vi "HostControl_Main.vi"() -> ()   [LabVIEW 2013]
uses:
  Support VIs/operationModes.ctl
  <vilib>/MakerHub/KinectOne/Private/Type Defs/BodyData.ctl
  <vilib>/MakerHub/KinectOne/Private/Type Defs/ClippedEdges.ctl
  <vilib>/MakerHub/KinectOne/Private/Type Defs/HandLeftConfidence.ctl
  <vilib>/MakerHub/KinectOne/Private/Type Defs/HandLeftState.ctl
  <vilib>/MakerHub/KinectOne/Private/Type Defs/HandRightConfidence.ctl
  <vilib>/MakerHub/KinectOne/Private/Type Defs/HandRightState.ctl
  Microsoft.Kinect
  <vilib>/MakerHub/KinectOne/Private/Type Defs/LeanTrackingState.ctl
  Messages.ctl
  Support VIs/messageTypes.ctl
  GainsTDef.ctl
  Support VIs/speeds.ctl
  PolarCoordTdef.ctl
  StopTDef.ctl
  Support VIs/setpointCluster.ctl
  <vilib>/MakerHub/PS4-Controller/Public/Open First Controller.vi
  <vilib>/MakerHub/KinectOne/Private/Initialize Image [Color].vi
  <vilib>/MakerHub/KinectOne/Private/kinectRead [ColorFrame].vi
  <vilib>/MakerHub/KinectOne/Private/kinectRead [BodyFrame].vi
  <vilib>/MakerHub/KinectOne/KinectOne.lvlib
  <vilib>/MakerHub/PS4-Controller/LMH-PS4.lvlib
panel:
  in  "colour mode (T = dist, F = sphere)":bool
  out "Detected Colour":u32(colorbox)
  out "Tracked?":bool
  in  "Forward Speed Limit [rad/s] (10 r/s)":dbl(knob)=2.995028509599303 scale=0.0..10.0
  out "Gains Closed":bool
  out "Setpoint Grtr Closed":bool
  out "Stopper Closed":bool
  out "Kinect Closed":bool
  out "Ctrl Event Loop Off":bool
  out "Controller Off":bool
  out "Hand Ctrl Closed":bool
  out "Message Sender Closed":bool
  in  "ControllerStop":bool
  out "Controller?":bool
  out "Toggle":bool
  in  "Cancel Button":bool
  out "TX":bool
  in  "bodyData":T1[](array[typedef])
  in  "Modulus SP":dbl=1.8
  in  "Reference Colour":u32(colorbox)
  in  "Argument SP":dbl
  out "index":i32
  in  "Operation Mode":T8=1 items=["TeleOp", "Desperate", "ColourMatch"]
  out "Image":T9(plugin-control)
  in  "Kd-Argument":dbl
  in  "Kc-Argument":dbl=0.3
  in  "Kd-Modulus":dbl
  in  "Kc-Modulus":dbl=0.5
  out "Mod":dbl
  out "Arg":dbl
  in  "IT'S TIME TO":bool
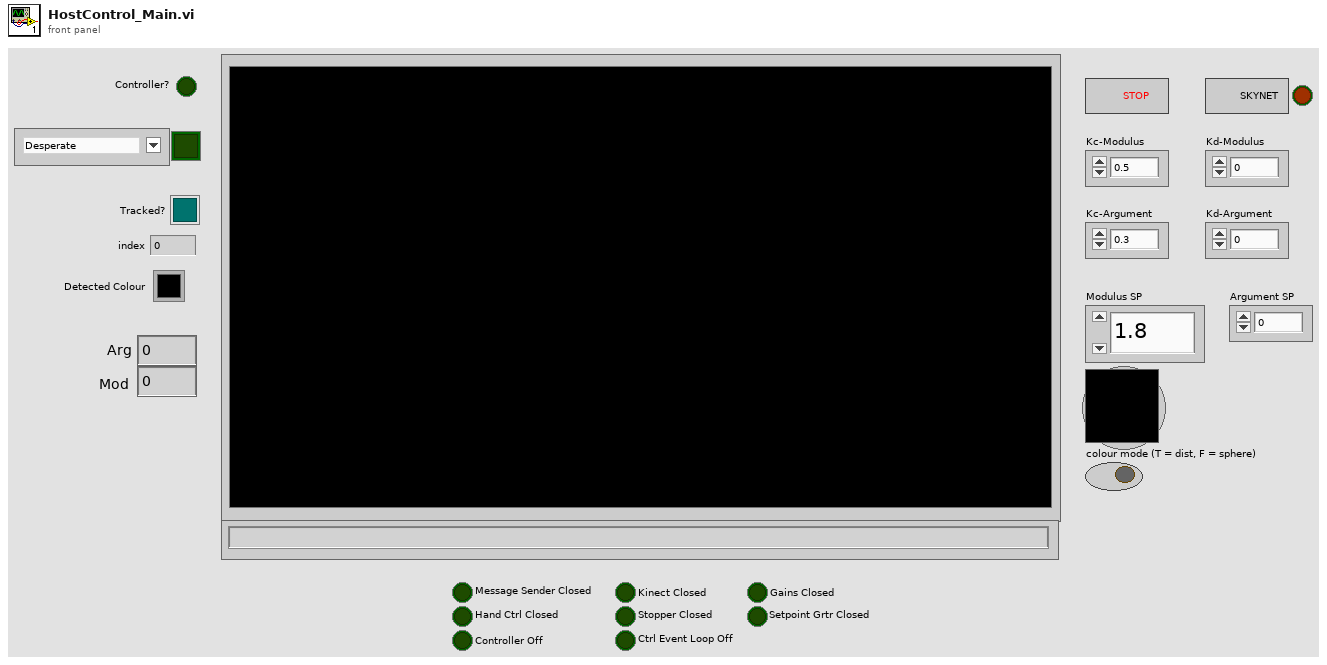
[diagram p1: front panel]
types:
  T1 = typedef "KinectOne.lvlib/BodyData.ctl" = cluster{"ClippedEdges":T2, "HandLeftConfidence":T3, "HandLeftState":T4, "HandRightConfidence":T5, "HandRightState":T6, "IsRestricted":bool, "IsTracked":bool, "JointOrientations":refnum<k24>, "Joints":refnum<k24>, "Lean":refnum<k24>, "LeanTrackingState":T7, "TrackingId":u64}
  T2 = typedef "KinectOne.lvlib/ClippedEdges.ctl" = enum16{"None", "Right", "Left", "Top", "Bottom"}
  T3 = typedef "KinectOne.lvlib/HandLeftConfidence.ctl" = enum16{"Low", "High"}
  T4 = typedef "KinectOne.lvlib/HandLeftState.ctl" = enum16{"Unknown", "NotTracked", "Open", "Closed", "Lasso"}
  T5 = typedef "KinectOne.lvlib/HandRightConfidence.ctl" = enum16{"Low", "High"}
  T6 = typedef "KinectOne.lvlib/HandRightState.ctl" = enum16{"Unknown", "NotTracked", "Open", "Closed", "Lasso"}
  T7 = typedef "KinectOne.lvlib/LeanTrackingState.ctl" = enum16{"NotTracked", "Inferred", "Tracked"}
  T8 = typedef "operationModes.ctl" = u16
  T9 = typedef "IMAQ Image.ctl" = refnum<image>
  T10 = typedef "GainsTDef.ctl" = cluster{"Kc-Modulus":dbl, "Kd-Modulus":dbl, "Kc-Argument":dbl, "Kd-Argument":dbl}
  T11 = typedef "Messages.ctl" = cluster{"message data":variant, "message type":T12}
  T12 = typedef "messageTypes.ctl" = enum16{"Speeds", "Stop", "PolarCoordinates", "Gains", "Setpoints"}
  T13 = typedef "KinectOne.lvlib/KinectSensor References.ctl" = cluster{"KinectSensor":refnum<k24>, "MultiSourceFrameReader":refnum<k24>, "BodyFrameDataInterface":refnum<k24>}
  T14 = typedef "LMH-PS4.lvlib/PS4 Controller Ref.ctl" = cluster{"Controller Ref":refnum<k1>, "PS4 Events Ref":refnum<event-registration>, "Worker Ref":refnum<vi>}
  T15 = typedef "StopTDef.ctl" = cluster{"stop":bool}
  T16 = typedef "speeds.ctl" = cluster{"left motor [rad/s]":dbl, "right motor [rad/s]":dbl}
  T17 = typedef "PolarCoordTdef.ctl" = cluster{"Argument":dbl, "Modulus":dbl, "trackedState":bool}
  T18 = typedef "KinectOne.lvlib/Joint Position.ctl" = cluster{"Camera Space":cluster{"X":dbl, "Y":dbl, "Z":dbl}, "Color Space":cluster{"X":dbl, "Y":dbl}, "Depth Space":cluster{"X":dbl, "Y":dbl}, "Tracking State":enum16{"NotTracked", "Inferred", "Tracked"}}
  T19 = typedef "setpointCluster.ctl" = cluster{"Modulus Setpoint":dbl, "Argument Setpoint":dbl}
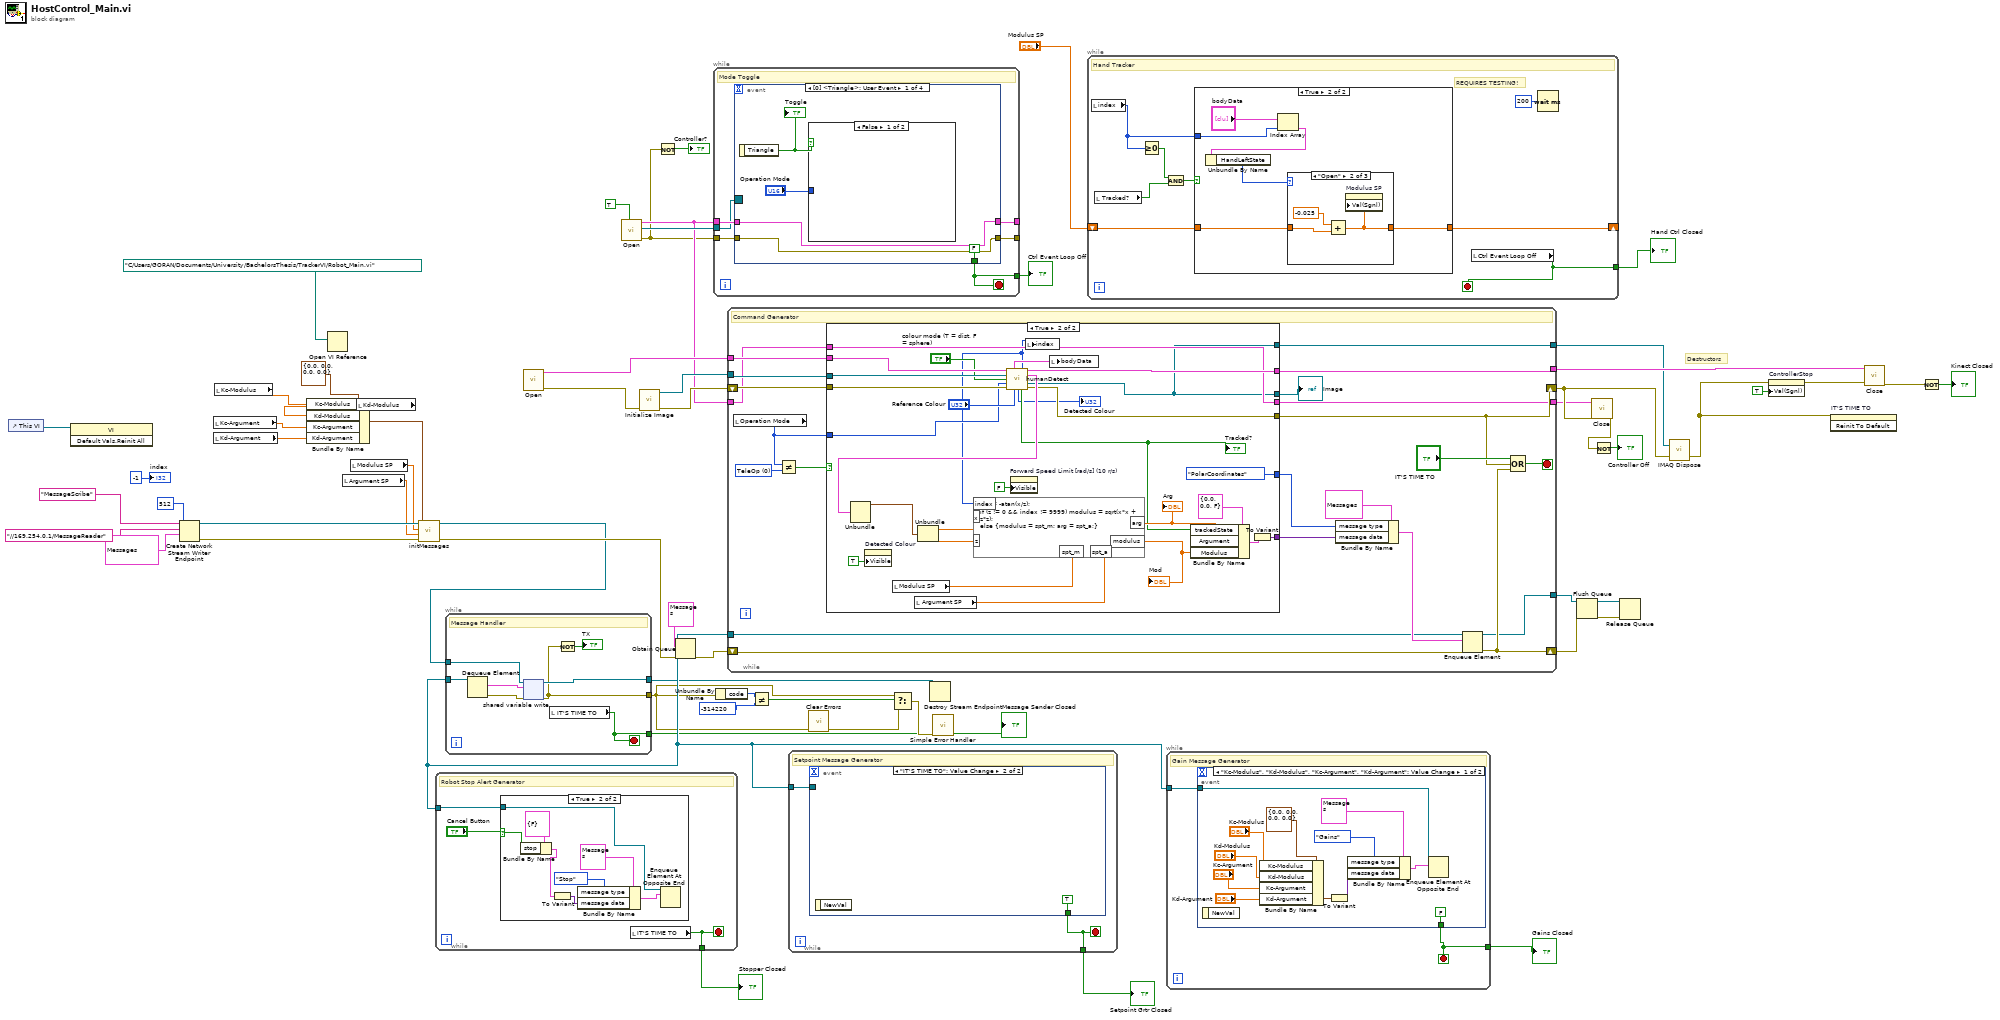
[diagram p0: block diagram]
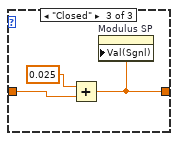
[diagram p4: hidden frame]
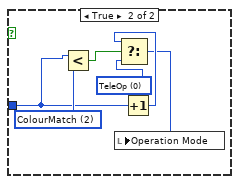
[diagram p5: hidden frame]
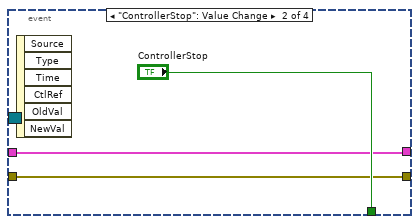
[diagram p6: hidden frame]
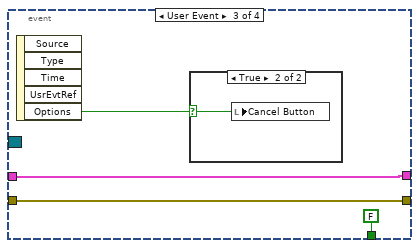
[diagram p7: hidden frame]
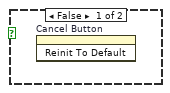
[diagram p8: hidden frame]
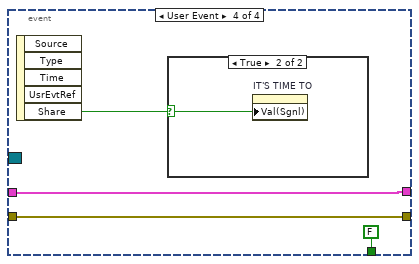
[diagram p9: hidden frame]
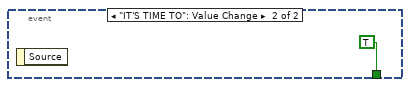
[diagram p12: hidden frame]
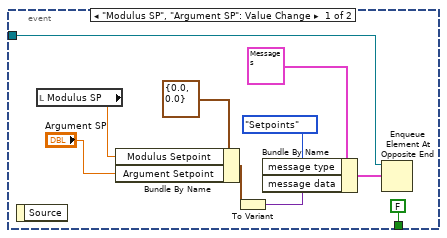
[diagram p13: hidden frame]
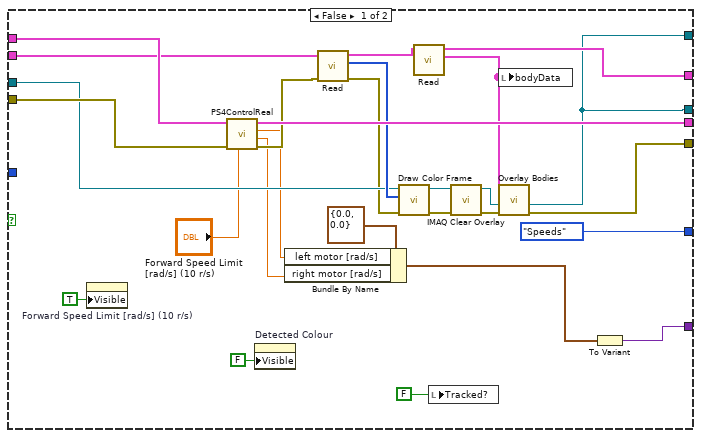
[diagram p14: hidden frame]
diagram:
  # "Destructors"
  n1 = control-ref of="This VI"() -> (w4:refnum<vi>)
  n2 = invoke class="VI" method="Default Vals.Reinit All"(reference=w4) -> ()  [unwired: 2 in, 3 out]
  n3 = Create Network Stream Writer Endpoint(7:512 ("writer buffer size"), 9:T11 {"message data"=variant, "message type"=enum."Setpoints"} ("message"), 10:"//169.254.0.1/MessageReader" ("reader url"), 11:"MessageScribe" ("writer name")) -> (0:w25:errorcluster, 3:w26:refnum<k21>)  [unwired: 3 in]
  n4 = local read "Kc-Argument"() -> (w29:dbl)
  n5 = local read "Kd-Argument"() -> (w28:dbl)
  n6 = local read "Kc-Modulus"() -> (w31:dbl)
  n7 = Open VI Reference(vi path=path "C:/Users/GORAN/Documents/University/BachelorsThesis/TrackerVI/Robot_Main.vi") -> ()  [unwired: 5 in, 2 out]
  n8 = local read "Argument SP"() -> (w23:dbl)
  n9 = local read "Modulus SP"() -> (w24:dbl)
  n10 = local read "Kd-Modulus"() -> (w30:dbl)
  n11 = Bundle By Name(cluster=T10 {"Kc-Modulus"=0.0, "Kd-Modulus"=0.0, "Kc-Argument"=0.0, "Kd-Argument"=0.0}, "Kc-Modulus"=w31, "Kd-Modulus"=w30, "Kc-Argument"=w29, "Kd-Argument"=w28) -> (w27:T10)
  n12 = call "initMessages.vi"("GainsCluster"=w27, "error in (no error)"=w25, "Argument Setpoint"=w23, "Modulus Setpoint"=w24, "writer name in"=w26) -> ("error out"=w22:errorcluster, "Refnum out"=w21:refnum<k21>)  [unwired: 5 in]
  n13 = call <vilib>:"Open.vi"() -> ("Error Out"=w60:errorcluster, "KinectSensor References out"=w52:T13)  [unwired: 10 in]
  n14 = call-poly <vilib>:"Open.vi"("Enable Events (T)"=TRUE) -> ("Error Out"=w20:errorcluster, "Event Registration Refnum"=w53:refnum<event-registration>, "PS4 Controller Ref"=w51:T14)  [unwired: 8 in]
  n15 = call-poly <vilib>:"Initialize Image.vi"("Error In"=w60) -> ("Error Out"=w59:errorcluster, "Color Image"=w58:T9)  [unwired: 9 in]
  n16 = Not(x=w20) -> (.not. x?=→"Controller?":bool)
  n17 = Obtain Queue(element data type=T11 {"message data"=variant, "message type"=enum."Stop"} ("message"), error in (no error)=w22) -> (queue out=w49:refnum<queue>, error out=w56:errorcluster)  [unwired: 3 in, 1 out]
  n18 = while {
    tunnel: w49 -> [w63]
    tunnel: [w61] -> w7
    stop <- w61 stop-if-true
    # "Robot Stop Alert Generator"
    n19 = case shown="True" "Cancel Button" {
      selector: "Cancel Button" -> [_ w66]
      tunnel: w63 -> [_ w67]
      frame False {
      }
      frame True {
        n20 = Bundle By Name(cluster=T15 {"stop"=FALSE} ("Cluster"), "stop"=w66) -> (w64:T15)
        n21 = To Variant(anything=w64) -> (Variant=w70:variant)
        n22 = Bundle By Name(cluster=T11 {"message data"=variant, "message type"=enum."Stop"} ("message"), "message type"=messageTypes."Stop", "message data"=w70) -> (w69:T11)
        n23 = Enqueue Element At Opposite End(queue=w67, element=w69) -> ()  [unwired: 2 in, 3 out]
      }
    }
    n24 = local read "IT'S TIME TO"() -> (w61:bool)
  }
  "Stopper Closed" <- w7
  n25 = while {
    tunnel: w49 -> [w79]
    tunnel: [w76] -> w34
    tunnel: [w75] -> w33
    tunnel: w21 -> [w73]
    tunnel: [w72] -> w8
    stop <- w72 stop-if-true
    # "Message Handler"
    n26 = Dequeue Element(queue=w79) -> (element=w78:T11, error out=w77:errorcluster)  [unwired: 2 in, 2 out]
    n27 = shared-variable-write(w73, w77, w78) -> (w76:refnum<k21>, w75:errorcluster)  [unwired: 1 in, 1 out]
    n28 = local read "IT'S TIME TO"() -> (w72:bool)
    n29 = Not(x=w75) -> (.not. x?=→"TX":bool)
  }
  "Message Sender Closed" <- w8
  n30 = while {
    tunnel: w53 -> [w83]
    tunnel: w20 -> [w84]
    tunnel: [w81] -> _
    tunnel: w51 -> [w85]
    tunnel: [w82] -> _
    tunnel: [w80] -> w9
    stop <- w80 stop-if-true
    # "Mode Toggle"
    n31 = event shown="[0] <Triangle>: User Event" {
      selector: w83 -> [_ _ _ _]
      dyn-events: _ -> [_ _ _ _]
      timeout: _ -> [_ _ _ _]
      tunnel: w85 -> [w88 w98 w102 w107]
      tunnel: w84 -> [w87 w97 w101 w106]
      tunnel: [w88 w98 w102 w107] -> w82
      tunnel: [w87 w97 w101 w106] -> w81
      tunnel: [FALSE ("ControllerStop") "ControllerStop" FALSE ("ControllerStop") FALSE ("ControllerStop")] -> w80
      event User Event {
        n32 = event-data() -> ("Triangle"=w90:bool)  [unwired: 1 in]
        "Toggle" <- w90
        n33 = case shown="False" w90 {
          tunnel: "Operation Mode" -> [_ w91]
          frame False {
          }
          frame True {
            w92 = T8 2 items=["TeleOp", "Desperate", "ColourMatch"] ("Operation Mode 2")
            w93 = T8 0 items=["TeleOp", "Desperate", "ColourMatch"] ("Operation Mode 2")
            n34 = Less?(x=w91, y=w92) -> (x < y?=w96:bool)
            n35 = Increment(x=w91) -> (x+1=w95:T8)
            n36 = Select(t=w95, s=w96, f=w93) -> (s? t:f=w94:T8)
            n37 = local write "Operation Mode"(w94) -> ()
          }
        }
      }
      event "ControllerStop": Value Change {
        n38 = event-data() -> ()  [unwired: 1 in, 6 out]
      }
      event User Event {
        n39 = event-data() -> ("Options"=w103:bool)  [unwired: 1 in, 4 out]
        n40 = case shown="True" w103 {
          selector: w103 -> [_ w104]
          frame False {
            n41 = invoke on="Cancel Button" class="Bool (strict)" method="Reinit To Default"() -> ()  [unwired: 3 in, 3 out]
          }
          frame True {
            n42 = local write "Cancel Button"(w104) -> ()
          }
        }
      }
      event User Event {
        n43 = event-data() -> ("Share"=w108:bool)  [unwired: 1 in, 4 out]
        n44 = case shown="True" w108 {
          selector: w108 -> [_ w109]
          frame False {
          }
          frame True {
            n45 = property on="IT'S TIME TO" class="Bool (strict)"("Val(Sgnl)"=w109) -> ()  [unwired: 2 in, 2 out]
          }
        }
      }
    }
  }
  "Ctrl Event Loop Off" <- w9
  n46 = Unbundle By Name(w33) -> ("code"=w42:i32)
  n47 = while {
    tunnel: w52 -> [w125]
    tunnel: w58 -> [w124]
    shift-right: [w123] -> w15
    shift-left: w59 -> [w122]
    tunnel: [w120] -> w57
    shift-right: [w127] -> w45
    shift-left: w56 -> [w128]
    tunnel: w49 -> [w126]
    tunnel: [w121] -> w54
    tunnel: [w111] -> w46
    tunnel: w51 -> [w118]
    tunnel: [w117] -> w14
    stop <- w131 stop-if-true
    w113 = T8 0 items=["TeleOp", "Desperate", "ColourMatch"] ("y")
    # "Command Generator"
    n48 = local read "Operation Mode"() -> (w114:T8)
    n49 = Not Equal?(x=w114, y=w113) -> (x != y?=w119:bool)
    n50 = case shown="True" w119 {
      tunnel: w125 -> [w155 w180]
      tunnel: w124 -> [w153 w179]
      tunnel: [w134 w177] -> w123
      tunnel: w122 -> [w157 w176]
      tunnel: [w135 w165] -> w121
      tunnel: [w138 w174] -> w120
      tunnel: w118 -> [w158 w167]
      tunnel: [w156 w167] -> w117
      tunnel: w114 -> [_ w171]
      tunnel: [messageTypes."Speeds" ("message type") messageTypes."PolarCoordinates" ("message type")] -> w116
      tunnel: [w146 w169] -> w115
      tunnel: [w135 w165] -> w110
      frame False {
        n51 = property on="Forward Speed Limit [rad/s] (10 r/s)" class="Knob (strict)"("Visible"=TRUE) -> ()  [unwired: 2 in, 2 out]
        n52 = call "PS4ControlReal.vi"("Forward Speed Limit [rad/s] (10.7 r/s)"="Forward Speed Limit [rad/s] (10 r/s)", "Error In"=w157, "PS4 Controller Ref In"=w158) -> ("Error Out"=w152:errorcluster, "right motor out"=w149:dbl, "left motor out"=w150:dbl, "PS4 Controller Ref Out"=w156:T14)  [unwired: 5 in]
        n53 = property on="Detected Colour" class="ColBox"("Visible"=FALSE) -> ()  [unwired: 2 in, 2 out]
        n54 = Bundle By Name(cluster=T16 {"left motor [rad/s]"=0.0, "right motor [rad/s]"=0.0}, "left motor [rad/s]"=w150, "right motor [rad/s]"=w149) -> (w147:T16)
        n55 = call-poly <vilib>:"Read.vi"("Error In"=w152, "KinectSensor References in"=w155) -> ("Error Out"=w151:errorcluster, "frameData"=w154:u32[], "KinectSensor References out"=w139:T13)  [unwired: 7 in]
        n56 = call <vilib>:"Draw Color Frame.vi"("Error In"=w151, "U32 Array"=w154, "Image"=w153) -> ("Error Out"=w137:errorcluster, "Image Out"=w141:T9)  [unwired: 7 in]
        n57 = call-poly <vilib>:"Read.vi"("KinectSensor References in"=w139) -> ("Body Data"=w133:T1[], "KinectSensor References out"=w138:T13)  [unwired: 8 in, 1 out]
        n58 = local write "Tracked?"(FALSE) -> ()
        n59 = call "IMAQ Clear Overlay"("error in (no error)"=w137, "Image"=w141) -> ("error out"=w136:errorcluster, "Image Out"=w140:T9)  [unwired: 8 in]
        n60 = local write "bodyData"(w133) -> ()
        n61 = call <vilib>:"Overlay Bodies.vi"("Error In"=w136, "Image"=w140, "Body Data"=w133) -> ("Error Out"=w134:errorcluster, "Image Out"=w135:T9)  [unwired: 7 in]
        n62 = To Variant(anything=w147) -> (Variant=w146:variant)
      }
      frame True {
        n63 = property on="Detected Colour" class="ColBox"("Visible"=TRUE) -> ()  [unwired: 2 in, 2 out]
        n64 = local read "Modulus SP"() -> (w175:dbl)
        n65 = local read "Argument SP"() -> (w173:dbl)
        n66 = call "humanDetect.vi"("KinectSensor References in"=w180, "Tracker"=w179, "colour mode (T = dist, F = sphere)"="colour mode (T = dist, F = sphere)", "Operation Mode"=w171, "Error In"=w176, "Reference Colour"="Reference Colour") -> ("Body Data"=w166:T1[], "index"=w159:i32, "KinectSensor References"=w174:T13, "Joint Position"=w178:T18, "Image"=w165:T9, "Averaged Colour"=→"Detected Colour":u32, "istracked"=w163:bool, "Error Out"=w177:errorcluster)  [unwired: 2 in]
        "Tracked?" <- w163
        n67 = Unbundle(w178) -> ("Camera Space"=w186:cluster{"X":dbl, "Y":dbl, "Z":dbl})  [unwired: 3 out]
        n68 = Unbundle(w186) -> ("X"=w184:dbl, "Z"=w183:dbl)  [unwired: 1 out]
        n69 = formula code="arg = -atan(x/z);\nif (z != 0 && index != 9999) modulus = sqrt(x*x + z*z);\nelse {modulus = spt_m; arg = spt_a;}"("x"=w184, "z"=w183, "spt_m"=w175, "spt_a"=w173, "index"=w159) -> ("arg"=w182:dbl, "modulus"=w181:dbl)
        "Arg" <- w182
        "Mod" <- w181
        n70 = property on="Forward Speed Limit [rad/s] (10 r/s)" class="Knob (strict)"("Visible"=FALSE) -> ()  [unwired: 2 in, 2 out]
        n71 = local write "index"(w159) -> ()
        n72 = local write "bodyData"(w166) -> ()
        n73 = Bundle By Name(cluster=T17 {"Argument"=0.0, "Modulus"=0.0, "trackedState"=FALSE}, "trackedState"=w163, "Argument"=w182, "Modulus"=w181) -> (w170:T17)
        n74 = To Variant(anything=w170) -> (Variant=w169:variant)
      }
    }
    "Image" <- w110
    n75 = Bundle By Name(cluster=T11 {"message data"=variant, "message type"=enum."Stop"} ("message"), "message type"=w116, "message data"=w115) -> (w129:T11)
    n76 = Enqueue Element(queue=w126, element=w129, error in (no error)=w128) -> (queue out=w111:refnum<queue>, error out=w127:errorcluster)  [unwired: 1 in, 1 out]
    n77 = Compound Arithmetic op=OR("IT'S TIME TO", w123, w127) -> (w131:bool)
  }
  n78 = Not Equal?(x=w42, y=-314220) -> (x != y?=w44:bool)
  n79 = while {
    tunnel: w49 -> [w188]
    tunnel: [w187] -> w5
    stop <- w187 stop-if-true
    # "Setpoint Message Generator"
    n80 = event shown="[1] \"IT'S TIME TO\": Value Change" {
      selector: _ -> [_ _]
      dyn-events: _ -> [_ _]
      timeout: _ -> [_ _]
      tunnel: w188 -> [w194 _]
      tunnel: [FALSE TRUE] -> w187
      event "Modulus SP", "Argument SP": Value Change {
        n81 = event-data() -> ()  [unwired: 1 in, 1 out]
        n82 = local read "Modulus SP"() -> (w192:dbl)
        n83 = Bundle By Name(cluster=T19 {"Modulus Setpoint"=0.0, "Argument Setpoint"=0.0} ("Setpoint Cluster"), "Modulus Setpoint"=w192, "Argument Setpoint"="Argument SP") -> (w193:T19)
        n84 = To Variant(anything=w193) -> (Variant=w196:variant)
        n85 = Bundle By Name(cluster=T11 {"message data"=variant, "message type"=enum."Stop"} ("message"), "message type"=messageTypes."Setpoints", "message data"=w196) -> (w195:T11)
        n86 = Enqueue Element At Opposite End(queue=w194, element=w195) -> ()  [unwired: 2 in, 3 out]
      }
      event "IT'S TIME TO": Value Change {
        n87 = event-data() -> ()  [unwired: 1 in, 1 out]
      }
    }
  }
  "Setpoint Grtr Closed" <- w5
  n88 = call <vilib>:"Clear Errors.vi"("error in (no error)"=w33) -> ("error out"=w41:errorcluster)  [unwired: 6 in]
  n89 = Select(t=w33, s=w44, f=w41) -> (s? t:f=w35:errorcluster)
  n90 = Destroy Stream Endpoint(11:w34) -> ()  [unwired: 1 in, 1 out]
  n91 = call <vilib>:"Simple Error Handler.vi"("error in (no error)"=w35) -> ()  [unwired: 4 in, 5 out]
  n92 = while {
    shift-right: [w201] -> _
    shift-left: "Modulus SP" -> [w203]
    tunnel: [w200] -> w1
    stop <- w200 stop-if-true
    # "REQUIRES TESTING!"
    # "Hand Tracker"
    n93 = local read "index"() -> (w204:i32)
    n94 = local read "Tracked?"() -> (w205:bool)
    n95 = Greater Or Equal To 0?(x=w204) -> (x >= 0?=w206:bool)
    n96 = And(x=w206, y=w205) -> (x .and. y?=w207:bool)
    n97 = case shown="True" w207 {
      tunnel: w204 -> [_ w214]
      tunnel: w203 -> [w208 w211]
      tunnel: [w208 w209] -> w201
      frame False {
      }
      frame True {
        n98 = Index Array(array="bodyData", index=w214) -> (element=w213:T1)
        n99 = Unbundle By Name(w213) -> ("HandLeftState"=w212:T4)
        n100 = case shown="\"Open\"" w212 {
          tunnel: w211 -> [w215 w217 w220]
          tunnel: [w215 w216 w219] -> w209
          frame "Unknown", Default {
          }
          frame "Open" {
            n101 = Add(x=-0.025, y=w217) -> (x+y=w216:dbl)
            n102 = property on="Modulus SP" class="DigNum (strict)"("Val(Sgnl)"=w216) -> ()  [unwired: 2 in, 2 out]
          }
          frame "Closed" {
            n103 = Add(x=0.025, y=w220) -> (x+y=w219:dbl)
            n104 = property on="Modulus SP" class="DigNum (strict)"("Val(Sgnl)"=w219) -> ()  [unwired: 2 in, 2 out]
          }
        }
      }
    }
    n105 = local read "Ctrl Event Loop Off"() -> (w200:bool)
    n106 = Wait (ms)(milliseconds to wait=u32 200) -> ()  [unwired: 1 out]
  }
  "Hand Ctrl Closed" <- w1
  n107 = while {
    tunnel: w49 -> [w223]
    tunnel: [w222] -> w6
    stop <- w222 stop-if-true
    # "Gain Message Generator"
    n108 = event shown="[0] \"Kc-Modulus\", \"Kd-Modulus\", \"Kc-Argument\", \"Kd-Argument\": Value Change" {
      selector: _ -> [_ _]
      dyn-events: _ -> [_ _]
      timeout: _ -> [_ _]
      tunnel: w223 -> [w226 _]
      tunnel: [FALSE TRUE] -> w222
      event "Kc-Modulus", "Kd-Modulus", "Kc-Argument", "Kd-Argument": Value Change {
        n109 = event-data() -> ()  [unwired: 1 in, 1 out]
        n110 = Bundle By Name(cluster=T10 {"Kc-Modulus"=0.0, "Kd-Modulus"=0.0, "Kc-Argument"=0.0, "Kd-Argument"=0.0}, "Kc-Modulus"="Kc-Modulus", "Kd-Modulus"="Kd-Modulus", "Kc-Argument"="Kc-Argument", "Kd-Argument"="Kd-Argument") -> (w230:T10)
        n111 = To Variant(anything=w230) -> (Variant=w229:variant)
        n112 = Bundle By Name(cluster=T11 {"message data"=variant, "message type"=enum."Stop"} ("message"), "message type"=messageTypes."Gains", "message data"=w229) -> (w227:T11)
        n113 = Enqueue Element At Opposite End(queue=w226, element=w227) -> ()  [unwired: 2 in, 3 out]
      }
      event "IT'S TIME TO": Value Change {
        n114 = event-data() -> ()  [unwired: 1 in, 1 out]
      }
    }
  }
  "Gains Closed" <- w6
  n115 = Flush Queue(queue=w46, error in (no error)=w45) -> (queue out=w48:refnum<queue>, error out=w47:errorcluster)  [unwired: 1 out]
  n116 = call <vilib>:"Close.vi"("Error In"=w15, "PS4 Controller Ref"=w14) -> ("Error Out"=w12:errorcluster)  [unwired: 9 in]
  n117 = Not(x=w12) -> (.not. x?=→"Controller Off":bool)
  n118 = Release Queue(queue=w48, error in (no error)=w47) -> ()  [unwired: 1 in, 3 out]
  n119 = call "IMAQ Dispose"("Image"=w54, "error in (no error)"=w15) -> ("error out"=w3:errorcluster)  [unwired: 4 in]
  n120 = property on="ControllerStop" class="Bool (strict)"(error in=w3, "Val(Sgnl)"=TRUE ("Value (Signaling)")) -> (error out=w17:errorcluster)  [unwired: 1 in, 1 out]
  n121 = invoke on="IT'S TIME TO" class="Bool (strict)" method="Reinit To Default"(error in=w3) -> ()  [unwired: 2 in, 3 out]
  n122 = call <vilib>:"Close.vi"("Error In"=w17, "KinectSensor References"=w57) -> ("Error Out"=w11:errorcluster)  [unwired: 9 in]
  n123 = Not(x=w11) -> (.not. x?=→"Kinect Closed":bool)
  "index" <- -1 ("index")
